vi "Test Variant Flatten Unflatten.vi"() -> ()   [LabVIEW 2016]
uses:
  <vilib>/measure/NI_MABase.lvlib
panel:
  out "VariantFlattenExp Error":errorcluster
  out "error out":errorcluster
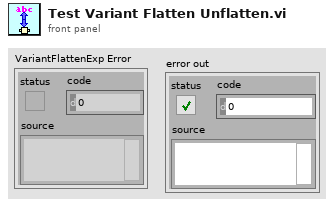
[diagram p1: front panel]
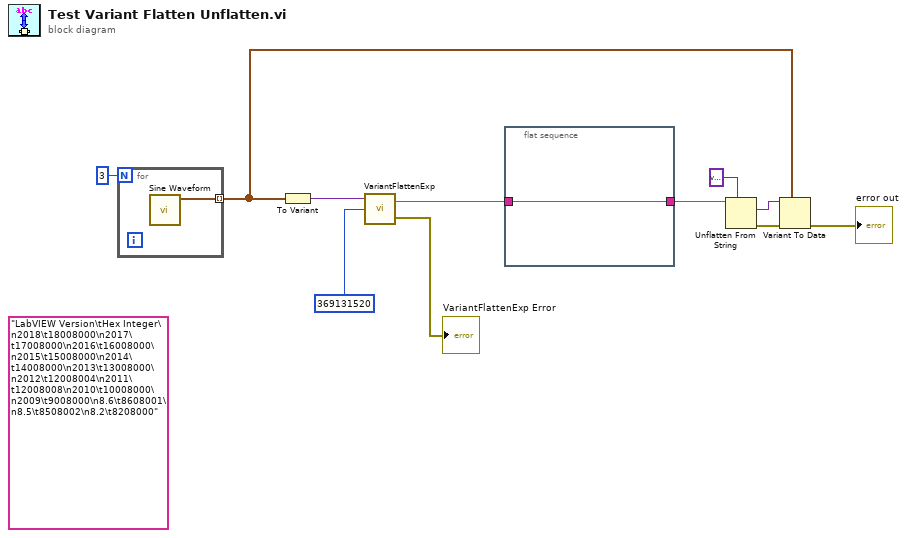
[diagram p0: block diagram]
diagram:
  (unwired) "LabVIEW Version\tHex Integer\n2018\t18008000\n2017\t17008000\n2016\t16008000\n2015\t15008000\n2014\t14008000\n2013\t13008000\n2012\t12008004\n2011\t12008008\n2010\t10008000\n2009\t9008000\n8.6\t8608001\n8.5\t8508002\n8.2\t8208000"
  n1 = for {
    N: 3 -> [_]
    tunnel: [w12] -> w2 mode=indexing
    n2 = call <vilib>:"Sine Waveform.vi"() -> ("signal out"=w12:waveform(dbl))  [unwired: 10 in, 1 out]
  }
  n3 = To Variant(anything=w2) -> (Variant=w1:variant)
  n4 = call <vilib>:"VariantFlattenExp.vi"("version"=u32 369131520, "variant"=w1) -> ("error out"=→"VariantFlattenExp Error":errorcluster, "data string"=w6:string)  [unwired: 1 in]
  n5 = flat-sequence {
    tunnel: w6 -> [w13]
    tunnel: [w13] -> w5
    frame #0 {
    }
  }
  n6 = Unflatten From String(type=variant, binary string=w5) -> (value=w8:variant, error out=w9:errorcluster)  [unwired: 3 in, 1 out]
  n7 = Variant To Data(error in=w9, type=w2, Variant=w8) -> (error out=→"error out":errorcluster)  [unwired: 1 out]
